vi "Add Package to SystemLink Feed.vi"() -> ()   [LabVIEW 2017]
doc: "This example shows how to upload and add a package to a SystemLink feed."
uses:
  SystemLink_Repo_API.lvlib
panel:
  out "Packages in the specified feed":string[][](table)
  in  "SystemLink Feed Name":string
  in  "Package Filepath":path
  in  "password":string
  in  "username":string
  in  "SystemLink server base URL":string="https://"
  # "SystemLink Server"
  # "Package to Add to SystemLink Feed"
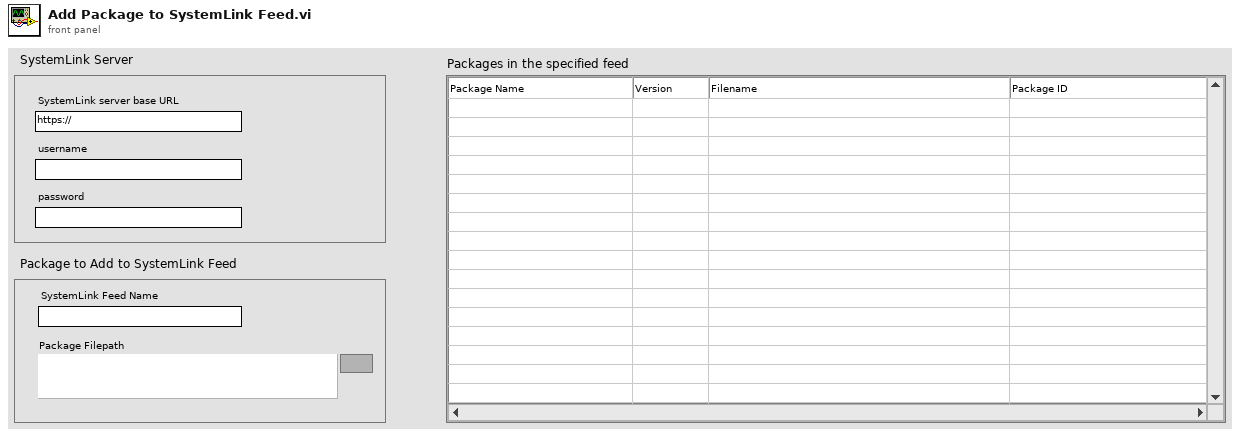
[diagram p1: front panel]
types:
  T1 = typedef "SystemLink_Repo_API.lvlib/systemlink repo.ctl" = cluster{"client handle out":T2, "SystemLink server base URL":string}
  T2 = typedef "LabVIEWHTTPClient.lvlib/ClientHandle.ctl" = refnum<k1>
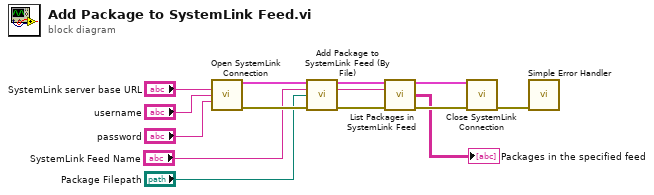
[diagram p0: block diagram]
diagram:
  n1 = call "Open SystemLink Connection.vi"("SystemLink server base URL"="SystemLink server base URL", "username"="username", "password"="password") -> ("SystemLink repo out"=w14:T1, "error out"=w13:errorcluster)  [unwired: 11 in]
  n2 = call "Add Package to SystemLink Feed (By File).vi"("SystemLink repo in"=w14, "feed name in"="SystemLink Feed Name", "package filepath"="Package Filepath", "error in (no error)"=w13) -> ("SystemLink repo out"=w6:T1, "feed name out"=w2:string, "error out"=w4:errorcluster)  [unwired: 8 in, 1 out]
  n3 = call "List Packages in SystemLink Feed.vi"("SystemLink repo in"=w6, "feed name in"=w2, "error in (no error)"=w4) -> ("SystemLink repo out"=w5:T1, "packages"=→"Packages in the specified feed":string[][], "error out"=w3:errorcluster)  [unwired: 9 in, 1 out]
  n4 = call "Close SystemLink Connection.vi"("SystemLink repo in"=w5, "error in (no error)"=w3) -> ("error out"=w9:errorcluster)  [unwired: 13 in]
  n5 = call <vilib>:"Simple Error Handler.vi"("error in (no error)"=w9) -> ()  [unwired: 4 in, 5 out]
